vi "追溯Global.vi"() -> ()   [LabVIEW 2020]
panel:
  out "DEVICE_ID":string
  out "USER_ID":string
  out "PRODUCT_ID":string
  out "CODE_ID":string
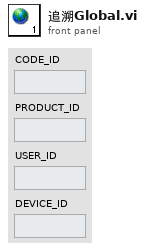
[diagram p1: front panel]
diagram:
